vi "cblas zdotu.vi"(5 "n":i32=-1, 6 "incy":i32=1, 7 "incx":i32=1, 10 "y":cdb[](array[numeric]), 11 "x":cdb[](array[numeric])) -> (0 "error":i32, 3 "zdotu":cdb)   [LabVIEW 2020, in "NI_AALBLAS.lvlib"]
uses:
  <vilib>/Analysis/NI_AALBLAS.lvlib
  <vilib>/Analysis/BLAS.llb/Operation_Conjugate.ctl
  <resource>/lvblas.dll
panel:
  # "void cblas_zdotu_sub(n, *x, incx, *y, incy, *zdotu)"
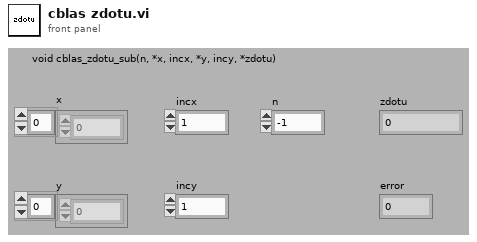
[diagram p1: front panel]
types:
  T1 = typedef "NI_AALBLAS.lvlib/Operation_Conjugate.ctl" = i32
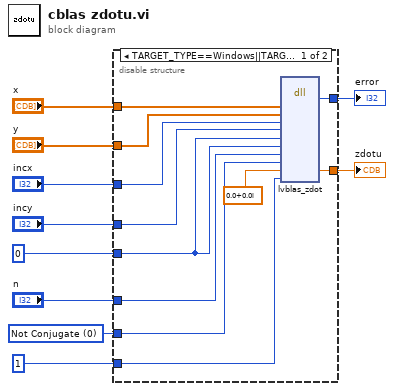
[diagram p0: block diagram]
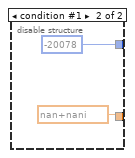
[diagram p2: hidden frame]
diagram:
  w5 = T1 0 items=["Not Conjugate", "Conjugate"] ("operation X")
  n1 = disable-structure shown="TARGET_TYPE==Windows||TARGET_TYPE==Unix||TARGET_TYPE==Mac||TARGET_TYPE==RT" {
    disable-tunnel: [w21 cdb nan+nani] -> w10
    disable-tunnel: "x" -> [w20 _]
    disable-tunnel: "y" -> [w19 _]
    disable-tunnel: "n" -> [w18 _]
    disable-tunnel: [w17 -20078 ("error")] -> w6
    disable-tunnel: w5 -> [w16 _]
    disable-tunnel: 0 -> [w15 _]
    disable-tunnel: "incx" -> [w13 _]
    disable-tunnel: "incy" -> [w12 _]
    disable-tunnel: 1 -> [w11 _]
    frame condition #0 (active) {
      n2 = dll-call lib="e:/builds/penguin/labview/branches/2020/dev/dist/resource/lvblas.*" fn="lvblas_zdot" ("CBLAS.dll:CxDotProdH")("X"=w20, "Y"=w19, "IncX"=w13, "IncY"=w12, "startX"=w15, "startY"=w15, "N"=w18, "OpX"=w16, "DotProd"=cdb 0.0+0.0i, "check"=w11) -> ("error"=w17:i32, "DotProd"=w21:cdb)  [unwired: 12 in, 2 out]
    }
    frame condition #1 {
    }
  }
  "error" <- w6
  "zdotu" <- w10
